vi "setAvailableShiftSpeeds.vi"(8 "error in (no error)":errorcluster, 10 "Available Shift Speeds":T1={"Vertical Shift Speeds"=[0.5250000357627869, 0.875, 1.5750000476837158, 2.9749999046325684, 5.775000095367432, 11.375, 22.57499885559082, 44.97500228881836], "Horizontal Shift Speeds"=[0.05, 1.0, 2.5]}, 11 "AndorIKonAcquisitor.lvclass in":refnum<class "AndorIKonAcquisitor.lvclass">) -> (0 "error out":errorcluster, 3 "AndorIKonAcquisitor.lvclass out":refnum<class "AndorIKonAcquisitor.lvclass">)   [LabVIEW 2011, in "Hardware.lvlib" / "Channels.lvlib" / "AndorIKonAcquisitor.lvclass"]
uses:
  AndorIKonAcquisitor.lvclass
  AndorIKonAcquisitor.lvclass/AndorIKonAcquisitor.ctl
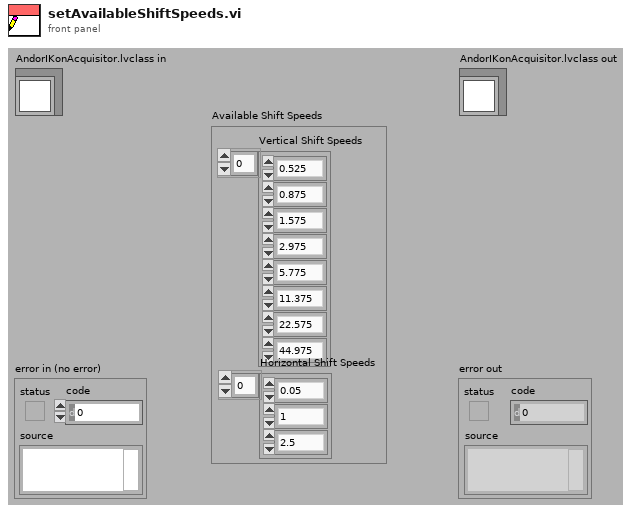
[diagram p1: front panel]
types:
  T1 = cluster{"Vertical Shift Speeds":dbl[], "Horizontal Shift Speeds":dbl[]}
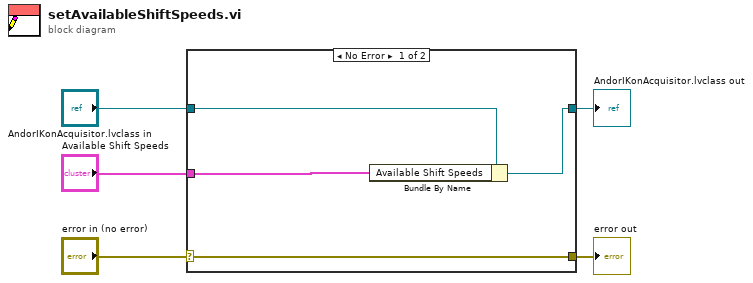
[diagram p0: block diagram]
diagram:
  n1 = case shown="No Error" "error in (no error)" {
    selector: "error in (no error)" -> [w9 w10]
    tunnel: [w9 w10] -> w4
    tunnel: [w7 w11] -> w2
    tunnel: "AndorIKonAcquisitor.lvclass in" -> [w8 w11]
    tunnel: "Available Shift Speeds" -> [w6 _]
    frame No Error {
      n2 = Bundle By Name(cluster=w8, "Available Shift Speeds"=w6) -> (w7:refnum<class "AndorIKonAcquisitor.lvclass">)
    }
    frame Error {
    }
  }
  "error out" <- w4
  "AndorIKonAcquisitor.lvclass out" <- w2
